vi "LSX Set Ext Value.vi"(8 "error in (no error)":errorcluster, 9 "lAValue":i32, 10 "lAName":i32, 11 "lLSID":i32) -> (0 "error out":errorcluster, 3 "function return":i32)   [LabVIEW 2018, in "Tango.lvlib"]
doc: "TANGOAPI int TANGOCALL LSX_SetExtValue (int lLSID, int lAName, int lAValue);"
uses:
  Tango.lvlib
  SubVIs/Tango_DLL.dll
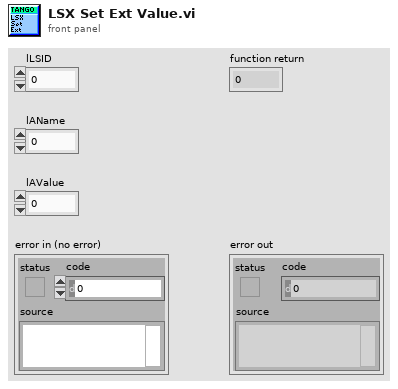
[diagram p1: front panel]
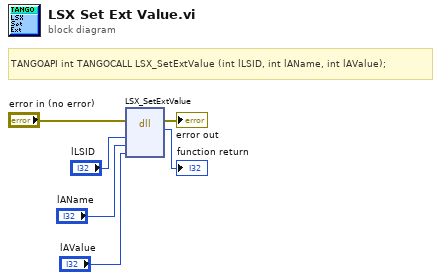
[diagram p0: block diagram]
diagram:
  # "TANGOAPI int TANGOCALL LSX_SetExtValue (int lLSID, int lAName, int lAValue);"
  n1 = dll-call lib="C:/Users/Familie/Documents/LabviewIX81/lib/TANGO Stage/SubVIs/Tango_DLL.*" fn="LSX_SetExtValue"(error in="error in (no error)", "lLSID"="lLSID", "lAName"="lAName", "lAValue"="lAValue") -> (error out=→"error out":errorcluster, →"function return":i32)  [unwired: 5 in, 1 out]
